vi "Do.vi"(8 "error in (no error)":errorcluster, 10 "Actor in":refnum<class "Actor.lvclass">, 11 "Configure Resume Trigger [RT] Msg":refnum<class "Configure Resume Trigger [RT] Msg.lvclass">) -> (0 "error out":errorcluster, 2 "Actor out":refnum<class "Actor.lvclass">)   [LabVIEW 2015, in "CS++Fgen.lvlib" / "Configure Resume Trigger [RT] Msg.lvclass"]
doc: "This VI delivers the message to the actor by calling the appropriate method(s) on the actor."
uses:
  Configure Resume Trigger [RT] Msg.lvclass
  <vilib>/ActorFramework/Actor/Actor.lvclass
  CS++Fgen/CS++Fgen.lvclass
  CSPP_Core/Actors/CS++PVMonitor Messages/CS++PVUpdate Msg/CS++PVUpdate Msg.lvclass/CS++PVUpdate Msg.ctl
  CSPP_Core/Classes/CS++ProcessVariables/ProcessVariable/PV.lvclass/PV.ctl
  Configure Resume Trigger [RT] Msg.lvclass/Configure Resume Trigger [RT] Msg.ctl
  CSPP_Core/Classes/CS++ProcessVariables/ProcessVariable/PV.lvclass
  CSPP_Core/Actors/CS++PVMonitor Messages/CS++PVUpdate Msg/CS++PVUpdate Msg.lvclass
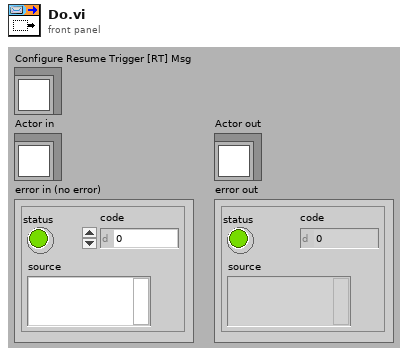
[diagram p1: front panel]
types:
  T1 = cluster{"Channel Name (\"\")":string, "Trigger Source (None)":string, "Trigger Slope (Positive)":i32}
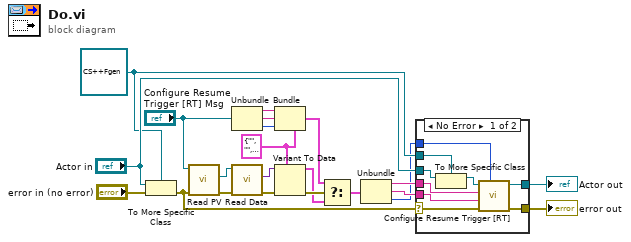
[diagram p0: block diagram]
diagram:
  w14 = T1 {"Channel Name (\"\")"="", "Trigger Source (None)"="", "Trigger Slope (Positive)"=0} ("Type")
  w18 = refnum<class "CS++Fgen.lvclass"> refnum ("Actor in")
  n1 = To More Specific Class(target class=w18, reference="Actor in", error in="error in (no error)") -> (error out=w7:errorcluster)  [unwired: 1 out]
  n2 = call "Read PV.vi"("error in (no error)"=w7, "CS++PVUpdate Msg in"="Configure Resume Trigger [RT] Msg") -> ("error out"=w17:errorcluster, "PV"=w13:refnum<class "PV.lvclass">)  [unwired: 7 in, 1 out]
  n3 = Unbundle ("Pre-Unbundler")("Configure Resume Trigger [RT] Msg") -> (w3:string, w2:string, w1:i32)
  n4 = call "Read Data.vi"("error in (no error)"=w17, "PV in"=w13) -> ("error out"=w11:errorcluster, "Data"=w12:variant)  [unwired: 7 in, 1 out]
  n5 = Bundle ("Pre-Bundler")(cluster=w14, "Channel Name (\"\")"=w3, "Trigger Source (None)"=w2, "Trigger Slope (Positive)"=w1) -> (w15:T1)
  n6 = Variant To Data(error in=w11, type=w14, Variant=w12) -> (data=w9:T1, error out=w16:errorcluster)
  n7 = Select ("MainSelect")(t=w15, s=w16, f=w9) -> (s? t:f=w10:T1)
  n8 = Unbundle ("Main-Unbundler")(w10) -> ("Channel Name (\"\")"=w6:string, "Trigger Source (None)"=w5:string, "Trigger Slope (Positive)"=w4:i32)
  n9 = case shown="No Error" w7 {
    selector: w7 -> [w29 w33]
    tunnel: [w31 w33] -> w21
    tunnel: [w30 w32] -> w20
    tunnel: "Actor in" -> [w28 w32]
    tunnel: w18 -> [w27 _]
    tunnel: w6 -> [w25 _]
    tunnel: w5 -> [w24 _]
    tunnel: w4 -> [w23 _]
    frame No Error {
      n10 = To More Specific Class(target class=w27, reference=w28) -> (specific class reference=w26:refnum<class "CS++Fgen.lvclass">)  [unwired: 1 in, 1 out]
      n11 = call "Configure Resume Trigger [RT].vi"("Trigger Slope (Positive)"=w23, "error in (no error)"=w29, "Trigger Source (None)"=w24, "Channel Name (\"\")"=w25, "CS++Fgen in"=w26) -> ("error out"=w31:errorcluster, "CS++Fgen out"=w30:refnum<class "CS++Fgen.lvclass">)  [unwired: 5 in]
    }
    frame Error {
    }
  }
  "error out" <- w21
  "Actor out" <- w20
